vi "New Worksheet.vi"(8 "error in (no error)":errorcluster, 11 "Worksheet.Ref":refnum<k24>) -> (0 "error out":errorcluster, 3 "worksheet out":refnum<class "worksheet.lvclass">)   [LabVIEW 2017, in "Excel_Specific.lvlib" / "worksheet.lvclass"]
uses:
  worksheet.lvclass
  C:/Users/Neo/Desktop/Dev_Tools_BR/LabVIEW_NPOI/src/lib/NPOI 2.1.1/NPOI.dll
  lib/NPOI 2.1.1/NPOI.dll
  worksheet.lvclass/worksheet.ctl
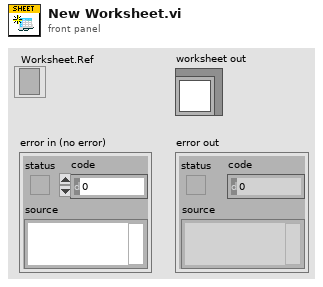
[diagram p1: front panel]
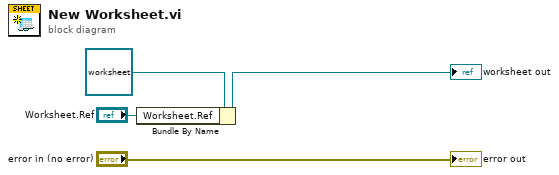
[diagram p0: block diagram]
diagram:
  n1 = Bundle By Name(cluster=refnum<class "worksheet.lvclass"> refnum ("worksheet in"), "Worksheet.Ref"="Worksheet.Ref") -> (→"worksheet out":refnum<class "worksheet.lvclass">)
  "error out" <- "error in (no error)"
